vi "Default Config File Path.vi"() -> (0 "Default config file name":path)   [LabVIEW 2020]
uses:
  <vilib>/Utility/sysdir.llb/System Directory Type.ctl
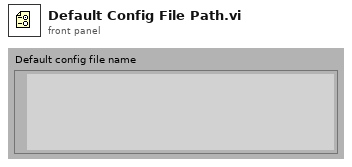
[diagram p1: front panel]
types:
  T1 = typedef "System Directory Type.ctl" = i32
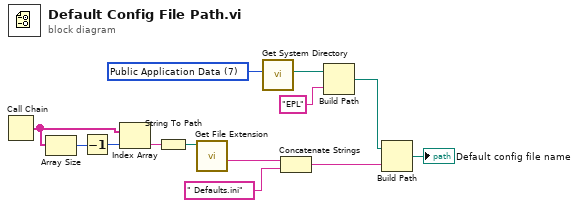
[diagram p0: block diagram]
diagram:
  w4 = T1 7 items=["User Home", "User Desktop", "User Documents", "User Application Data", "User Preferences", "User Temporary", "Public Documents", "Public Application Data", "Public Preferences", "System Core Libraries", "System Installed Libraries", "Application Files", "Boot Volume Root"] ("system directory type")
  n1 = Call Chain() -> (call chain=w13:string[])
  n2 = Array Size(array=w13) -> (size(s)=w12:i32)
  n3 = Decrement(x=w12) -> (x-1=w10:i32)
  n4 = Index Array(array=w13, index=w10) -> (element=w8:string)
  n5 = String To Path(string=w8) -> (path=w9:path)
  n6 = call <vilib>:"Get File Extension.vi"("file"=w9) -> ("filename without extension"=w7:string)  [unwired: 6 in, 4 out]
  n7 = call <vilib>:"Get System Directory.vi"("system directory type"=w4) -> ("system directory"=w3:path)  [unwired: 10 in]
  n8 = Concatenate Strings(w7, " Defaults.ini" ("string")) -> (w5:string)
  n9 = Build Path(base path=w3, name or relative path="EPL") -> (appended path=w2:path)
  n10 = Build Path(base path=w2, name or relative path=w5) -> (appended path=→"Default config file name":path)
